vi "LIN_EPA aktiv setzen.vi"(8 "error in (no error)":errorcluster caption="Fehler (Eingang, kein Fehler)", 11 "Anzahl aktiv":i32) -> (0 "error out":errorcluster caption="Fehler (Ausgang)", 3 "Aktiv":bool[][](array[boolean]))   [LabVIEW 2020, in "Linearisierung v2.lvlib"]
uses:
  Linearisierung v2.lvlib
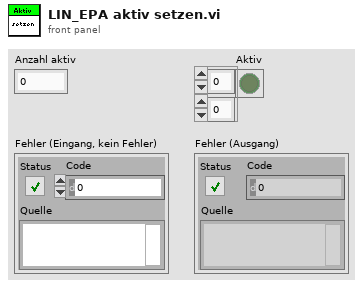
[diagram p1: front panel]
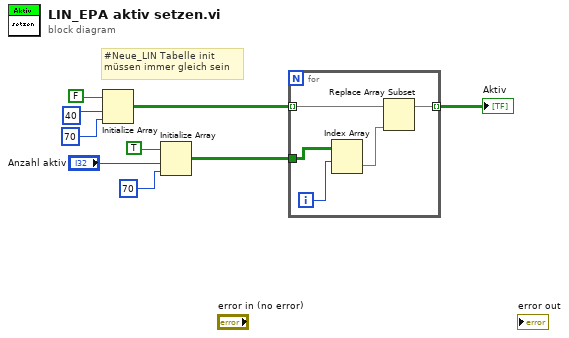
[diagram p0: block diagram]
diagram:
  # "#Neue_LIN Tabelle init\nmüssen immer gleich sein"
  n1 = Initialize Array(FALSE, 40 ("Dimension"), 70 ("Dimension")) -> (w2:bool[][])
  n2 = Initialize Array(TRUE, "Anzahl aktiv", 70 ("Dimension")) -> (w4:bool[][])
  n3 = for {
    tunnel: w4 -> [w12]
    tunnel: w2 -> [w14] mode=indexing
    tunnel: [w13] -> w3 mode=indexing
    i -> [w10]
    n4 = Index Array(array=w12, index (row)=w10) -> (element=w11:bool[])  [unwired: 1 in]
    n5 = Replace Array Subset(array=w14, new element=w11) -> (w13:bool[])  [unwired: 1 in]
  }
  "Aktiv" <- w3
